vi "Read keeper_plays.vi"(8 "error in (no error)":errorcluster, 11 "Playbook in":refnum<class "Playbook.lvclass">) -> (0 "error out":errorcluster, 2 "keeper_plays":T1, 3 "Playbook out":refnum<class "Playbook.lvclass">)   [LabVIEW 2021, in "Playbook.lvclass"]
uses:
  Playbook.lvclass
  keeper_plays.ctl
  Play_class/Play.lvclass
  TestPlay_class/TestPlay.lvclass
  HaltPlay_class/HaltPlay.lvclass
  KeeperPlay_class/KeeperPlay.lvclass
  TimeoutPlay_class/TimeoutPlay.lvclass
  ZigZagPlay_class/ZigZagPlay.lvclass
  GoToPlay_class/GoToPlay.lvclass
  BallPlacementPlay_class/BallPlacementPlay.lvclass
  BallPlacementAllyPlay_class/BallPlacementAllyPlay.lvclass
  SimpleBallPlacementAllyPlay_class/SimpleBallPlacementAllyPlay.lvclass
  Playbook.lvclass/Playbook.ctl
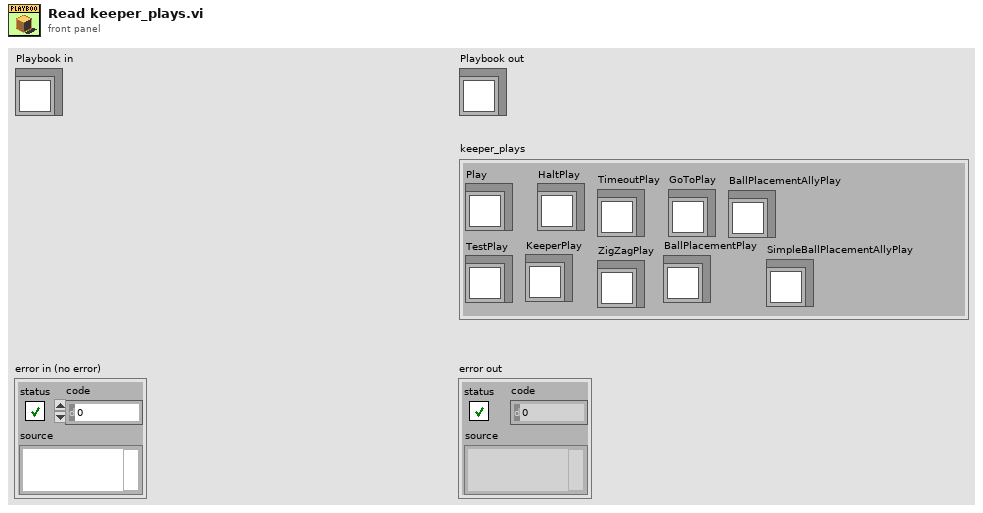
[diagram p1: front panel]
types:
  T1 = typedef "keeper_plays.ctl" = cluster{"Play":refnum<class "Play.lvclass">, "TestPlay":refnum<class "TestPlay.lvclass">, "HaltPlay":refnum<class "HaltPlay.lvclass">, "KeeperPlay":refnum<class "KeeperPlay.lvclass">, "TimeoutPlay":refnum<class "TimeoutPlay.lvclass">, "ZigZagPlay":refnum<class "ZigZagPlay.lvclass">, "GoToPlay":refnum<class "GoToPlay.lvclass">, "BallPlacementPlay":refnum<class "BallPlacementPlay.lvclass">, "BallPlacementAllyPlay":refnum<class "BallPlacementAllyPlay.lvclass">, "SimpleBallPlacementAllyPlay":refnum<class "SimpleBallPlacementAllyPlay.lvclass">}
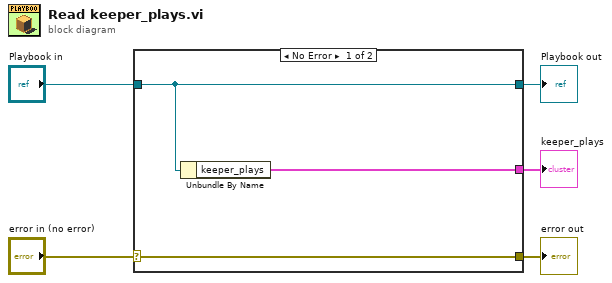
[diagram p0: block diagram]
diagram:
  n1 = case shown="No Error" "error in (no error)" {
    selector: "error in (no error)" -> [w8 w9]
    tunnel: [w8 w9] -> w4
    tunnel: [w7 w10] -> w2
    tunnel: "Playbook in" -> [w7 w10]
    tunnel: [w6 _] -> w1
    frame No Error {
      n2 = Unbundle By Name(w7) -> ("keeper_plays"=w6:T1)
    }
    frame Error {
    }
  }
  "error out" <- w4
  "Playbook out" <- w2
  "keeper_plays" <- w1
